vi "Read configuration.vi"(8 "error in (no error)":errorcluster, 11 "Start in":refnum<class "start.lvclass">) -> (0 "error out":errorcluster, 2 "configuration":string, 3 "Start out":refnum<class "start.lvclass">)   [LabVIEW 2016, in "Commands.lvlib" / "start.lvclass"]
uses:
  start.lvclass
  start.lvclass/start.ctl
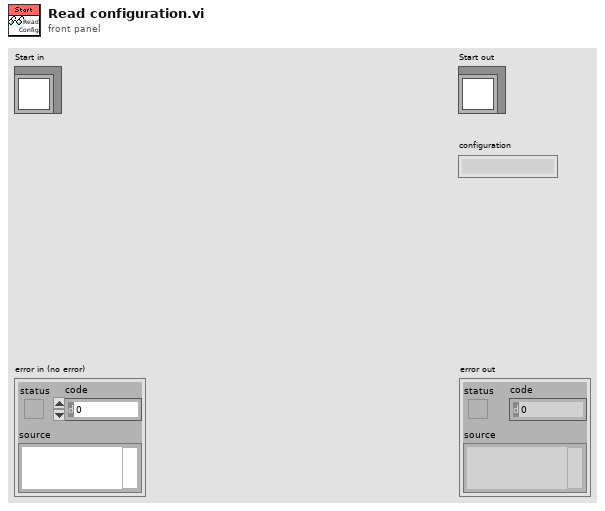
[diagram p1: front panel]
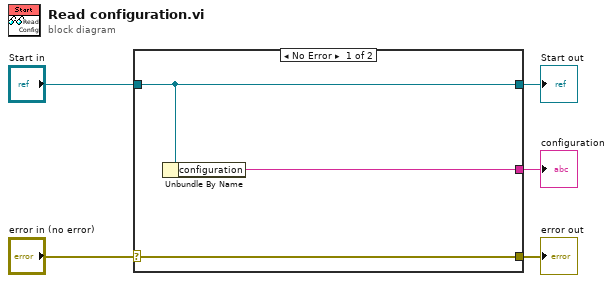
[diagram p0: block diagram]
diagram:
  n1 = case shown="No Error" "error in (no error)" {
    selector: "error in (no error)" -> [w8 w9]
    tunnel: [w8 w9] -> w4
    tunnel: [w7 w10] -> w2
    tunnel: "Start in" -> [w7 w10]
    tunnel: [w6 _] -> w1
    frame No Error {
      n2 = Unbundle By Name(w7) -> ("configuration"=w6:string)
    }
    frame Error {
    }
  }
  "error out" <- w4
  "Start out" <- w2
  "configuration" <- w1
